vi "Collect information from UI to run measurement.vi"(8 "error in (no error)":errorcluster, 11 "Measurement UI in":refnum<class "Controller UI.lvclass">) -> (0 "error out":errorcluster, 1 "Show UI?":bool, 2 "Device Names":string[](array[string]), 3 "Measurement UI out":refnum<class "Controller UI.lvclass">, 4 "String":string, 5 "Measurement Name":string)   [LabVIEW 2016, in "Controller UI.lvlib" / "Controller UI.lvclass"]
uses:
  <userlib>/Common Components/Controller UI/Controller UI.lvclass
  <userlib>/Common Components/Controller UI/Controller UI.lvclass/Controller UI.ctl
  <userlib>/Common Components/Controller UI/Accessors/Read Measurement.vi
  <userlib>/Common Components/Controller UI/Accessors/Read Temperature Controller.vi
  <userlib>/Common Components/Controller UI/Accessors/Read Show FP_.vi
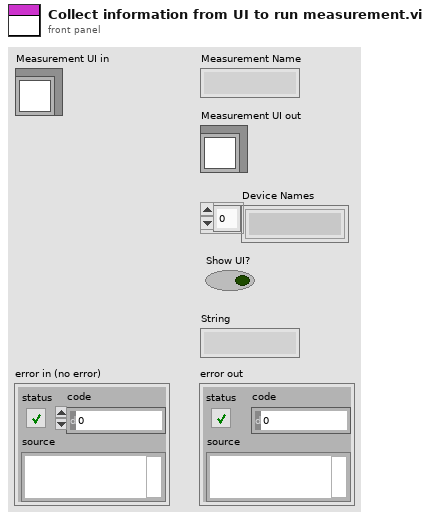
[diagram p1: front panel]
types:
  T1 = enum8{"Enabled", "Disabled", "Disabled and Grayed Out"}
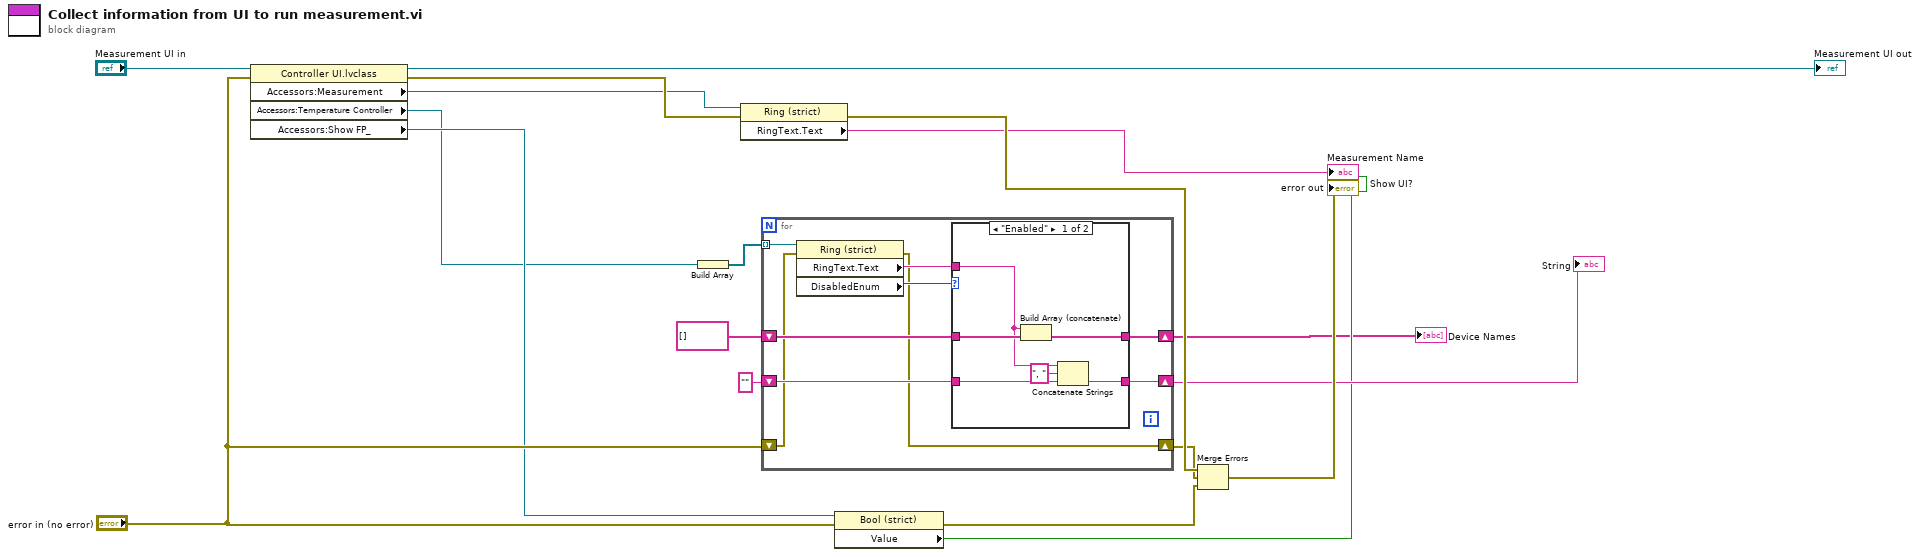
[diagram p0: block diagram]
diagram:
  n1 = property class="Controller UI.lvclass"(reference="Measurement UI in", error in="error in (no error)") -> (reference out=→"Measurement UI out":refnum<class "Controller UI.lvclass">, error out=w13:errorcluster, "Accessors:Measurement"=w12:refnum<vi>, "Accessors:Temperature Controller"=w1:refnum<vi>, "Accessors:Show FP_"=w11:refnum<vi>)
  n2 = Build Array(w1) -> (w4:refnum<vi>[])
  n3 = property class="Ring (strict)"(reference=w12, error in=w13) -> (error out=w17:errorcluster, "RingText.Text"=→"Measurement Name":string)  [unwired: 1 out]
  n4 = for {
    shift-right: [w24] -> w3
    shift-left: string[] [] ("Device Names") -> [w23]
    tunnel: w4 -> [w27] mode=indexing
    shift-right: [w22] -> w8
    shift-left: "" -> [w21]
    shift-right: [w20] -> w15
    shift-left: "error in (no error)" -> [w19]
    n5 = property class="Ring (strict)"(reference=w27, error in=w19) -> (error out=w20:errorcluster, "RingText.Text"=w25:string, "DisabledEnum"=w26:T1)  [unwired: 1 out]
    n6 = case shown="\"Enabled\"" w26 {
      tunnel: w25 -> [w29 _]
      tunnel: [w33 w35] -> w24
      tunnel: w23 -> [w32 w35]
      tunnel: [w31 w34] -> w22
      tunnel: w21 -> [w30 w34]
      frame "Enabled" {
        n7 = Build Array (concatenate)(w29, w32) -> (w33:string[])
        n8 = Concatenate Strings(w29, ", " ("string"), w30) -> (w31:string)
      }
      frame "Disabled", Default {
      }
    }
  }
  "String" <- w8
  "Device Names" <- w3
  n9 = property class="Bool (strict)"(reference=w11, error in="error in (no error)") -> (error out=w16:errorcluster, "Value"=→"Show UI?":bool)  [unwired: 1 out]
  n10 = Merge Errors(w17, w15, w16) -> (→"error out":errorcluster)
